vi "Main.vi"(8 "error in (no error)":errorcluster, 11 "Stop notifier":refnum<notifier>) -> (0 "error out":errorcluster)   [LabVIEW 2017, in "Error.lvlib"]
doc: "Module main"
uses:
  Error.lvlib
  ctl/StateData.ctl
  ctl/MainStates.ctl
  ctl/ErrorInfo.ctl
  <vilib>/ErrorRing/Error Ring.xnode
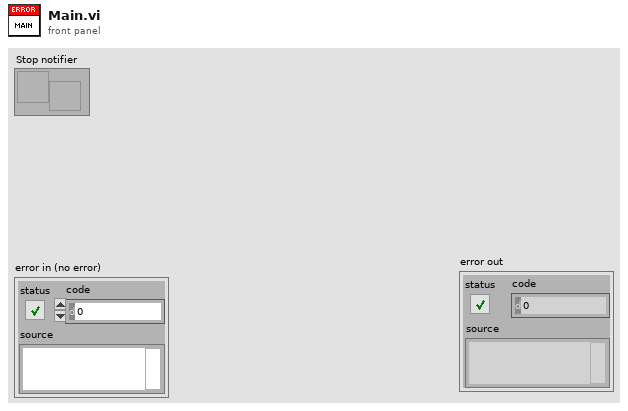
[diagram p1: front panel]
types:
  T1 = typedef "Error.lvlib/StateData.ctl" = cluster{"Blank":dbl}
  T2 = typedef "Error.lvlib/ErrorInfo.ctl" = cluster{"error in":errorcluster, "Text":string, "From":string, "Kill":bool}
  T3 = typedef "Error.lvlib/MainStates.ctl" = enum16{"Timeout", "Error", "Exit", "Init", "ClassError", "LogError", "Shutdown", "Warning"}
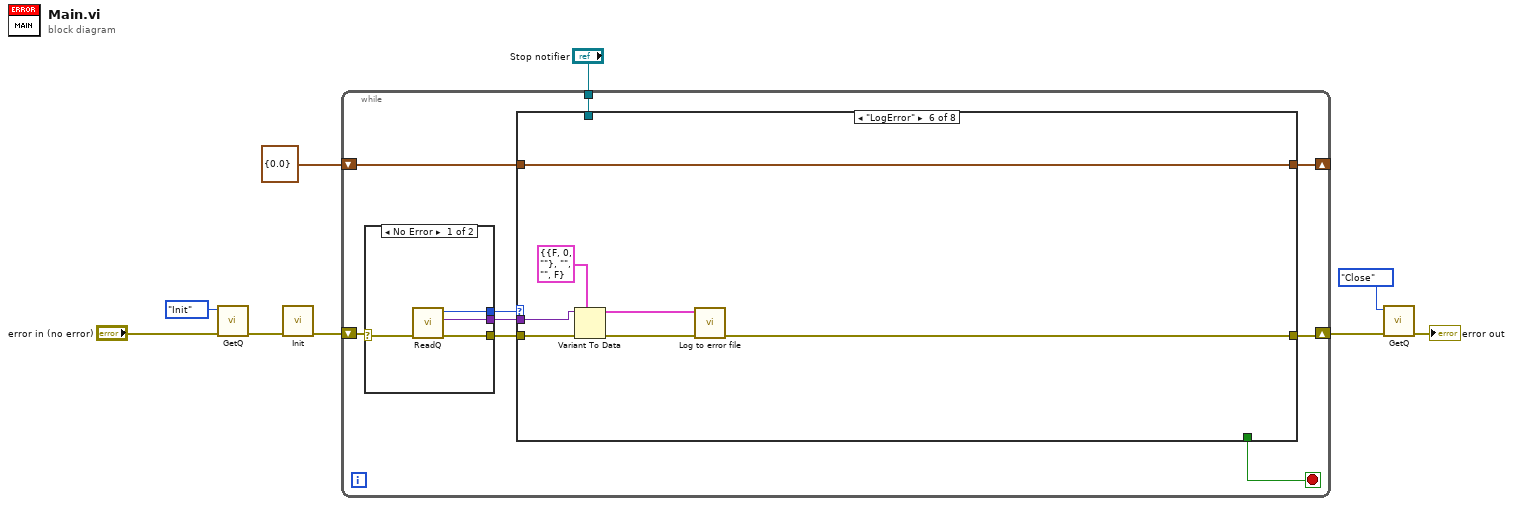
[diagram p0: block diagram]
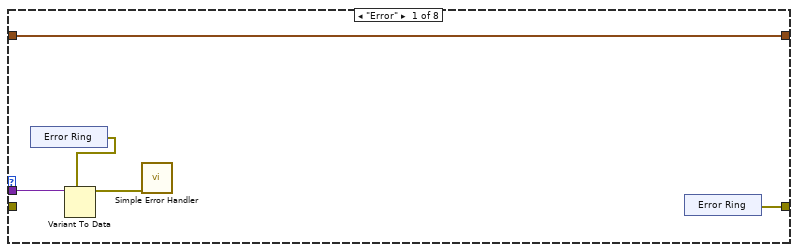
[diagram p2: hidden frame]
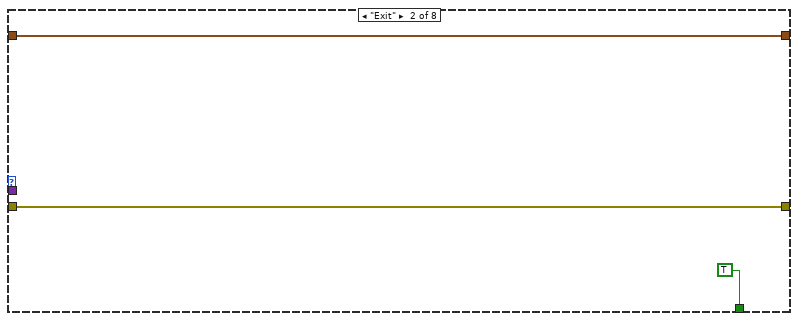
[diagram p3: hidden frame]
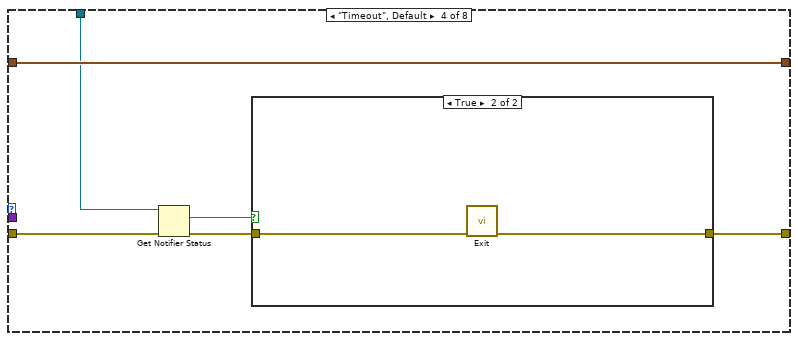
[diagram p5: hidden frame]
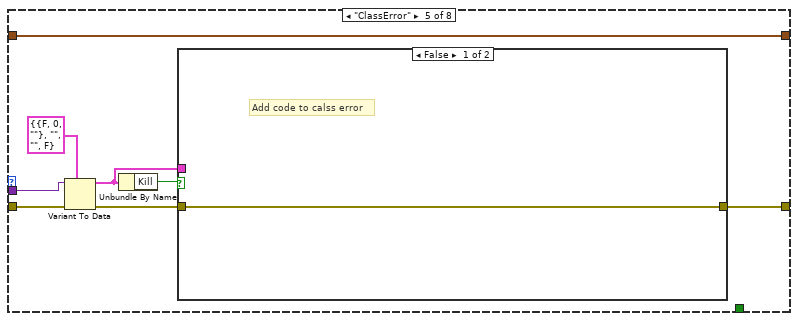
[diagram p7: hidden frame]
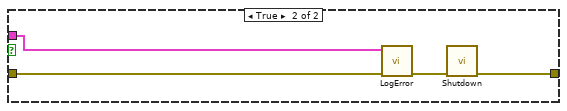
[diagram p8: hidden frame]
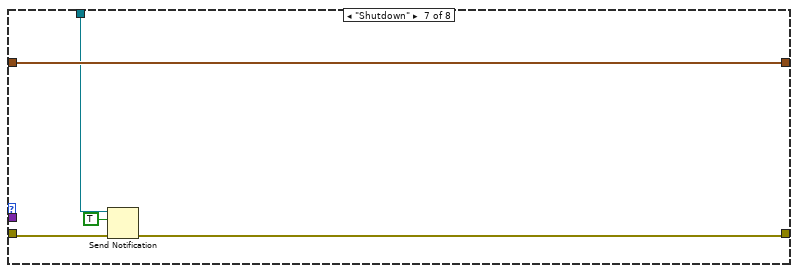
[diagram p9: hidden frame]
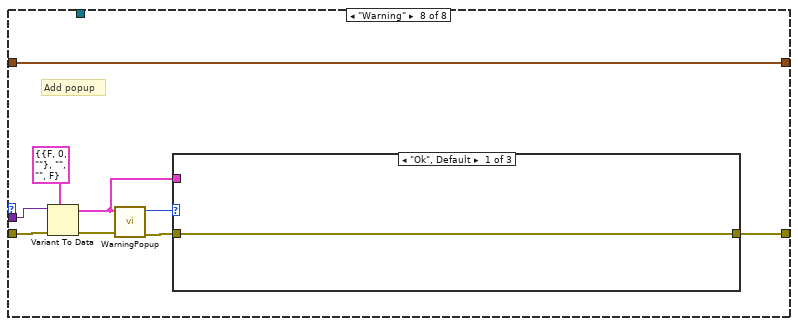
[diagram p10: hidden frame]
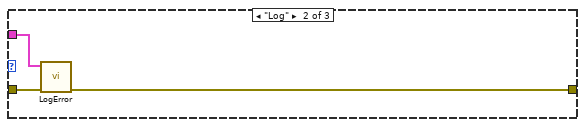
[diagram p11: hidden frame]
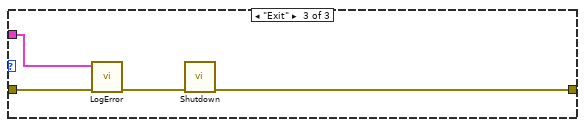
[diagram p12: hidden frame]
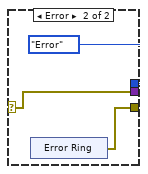
[diagram p13: hidden frame]
diagram:
  n1 = call "GetQ.vi"("error in (no error)"="error in (no error)", "Mode (Get)"=enum16{"Get", "Close", "Init"}."Init") -> ("error out"=w2:errorcluster)  [unwired: 8 in, 1 out]
  n2 = call "Init.vi"("error in (no error)"=w2) -> ("error out"=w1:errorcluster)  [unwired: 10 in]
  n3 = while {
    shift-right: [w14] -> w6
    shift-left: w1 -> [w18]
    shift-right: [w11] -> _
    shift-left: T1 {"Blank"=0.0} ("Cluster") -> [w12]
    tunnel: "Stop notifier" -> [w10]
    stop <- w13 stop-if-true
    n4 = case shown="No Error" w18 {
      selector: w18 -> [w85 w87]
      tunnel: [w84 MainStates."Error" ("State")] -> w17
      tunnel: [w83 w87] -> w16
      tunnel: [w82 w86] -> w15
      frame No Error {
        n5 = call "ReadQ.vi"("error in (no error)"=w85) -> ("error out"=w82:errorcluster, "Variant"=w83:variant, "State"=w84:T3)  [unwired: 8 in]
      }
      frame Error {
        n6 = xnode "Error Ring"() -> ("error out"=w86:errorcluster)
      }
    }
    n7 = case shown="\"LogError\"" w17 {
      tunnel: w16 -> [w23 _ _ _ w45 w56 _ w71]
      tunnel: w15 -> [_ w28 w30 w35 w46 w57 w63 w70]
      tunnel: [w22 w28 w30 w32 w41 w54 w60 w65] -> w14
      tunnel: [_ TRUE _ _ _ _ _ _] -> w13
      tunnel: w12 -> [w19 w26 w29 w36 w47 w59 w64 w73]
      tunnel: [w19 w26 w29 w36 w47 w59 w64 w73] -> w11
      tunnel: w10 -> [_ _ _ w34 _ _ w62 _]
      frame "Error" {
        n8 = xnode "Error Ring"() -> ("error out"=w21:errorcluster)
        n9 = Variant To Data(type=w21, Variant=w23) -> (data=w20:errorcluster)  [unwired: 1 in, 1 out]
        n10 = call <vilib>:"Simple Error Handler.vi"("error in (no error)"=w20) -> ()  [unwired: 4 in, 5 out]
        n11 = xnode "Error Ring"() -> ("error out"=w22:errorcluster)
      }
      frame "Exit" {
      }
      frame "Init" {
      }
      frame "Timeout", Default {
        n12 = Get Notifier Status(notifier=w34, error in (no error)=w35) -> (current notification=w33:bool, error out=w31:errorcluster)  [unwired: 3 out]
        n13 = case shown="True" w33 {
          tunnel: [w37 w38] -> w32
          tunnel: w31 -> [w37 w39]
          frame False {
          }
          frame True {
            n14 = call "Exit.vi"("error in (no error)"=w39) -> ("error out"=w38:errorcluster)  [unwired: 10 in]
          }
        }
      }
      frame "ClassError" {
        n15 = Variant To Data(error in=w46, type=T2 {"error in"={"status"=FALSE, "code"=0, "source"=""}, "Text"="", "From"="", "Kill"=FALSE} ("Error info"), Variant=w45) -> (data=w40:T2, error out=w42:errorcluster)
        n16 = Unbundle By Name(w40) -> ("Kill"=w43:bool)
        n17 = case shown="False" w43 {
          tunnel: w42 -> [w48 w50]
          tunnel: [w48 w52] -> w41
          tunnel: w40 -> [_ w49]
          frame False {
            # "Add code to calss error"
          }
          frame True {
            n18 = call "LogError.vi"("error in (no error)"=w50, "Error info"=w49) -> ("error out"=w51:errorcluster)  [unwired: 9 in]
            n19 = call "Shutdown.vi"("error in (no error)"=w51) -> ("error out"=w52:errorcluster)  [unwired: 10 in]
          }
        }
      }
      frame "LogError" {
        n20 = Variant To Data(error in=w57, type=T2 {"error in"={"status"=FALSE, "code"=0, "source"=""}, "Text"="", "From"="", "Kill"=FALSE} ("Error info"), Variant=w56) -> (data=w53:T2, error out=w55:errorcluster)
        n21 = call "Log to error file.vi"("error in (no error)"=w55, "Error info"=w53) -> ("error out"=w54:errorcluster)  [unwired: 9 in]
      }
      frame "Shutdown" {
        n22 = Send Notification(notification=TRUE, notifier=w62, error in (no error)=w63) -> (error out=w60:errorcluster)  [unwired: 1 out]
      }
      frame "Warning" {
        # "Add popup"
        n23 = Variant To Data(error in=w70, type=T2 {"error in"={"status"=FALSE, "code"=0, "source"=""}, "Text"="", "From"="", "Kill"=FALSE} ("Error info"), Variant=w71) -> (data=w66:T2, error out=w69:errorcluster)
        n24 = call "WarningPopup.vi"("error in (no error)"=w69, "Error info"=w66) -> ("error out"=w67:errorcluster, "Select"=w68:enum16{"Ok", "Log", "Exit"})  [unwired: 8 in]
        n25 = case shown="\"Ok\", Default" w68 {
          tunnel: w67 -> [w74 w77 w81]
          tunnel: w66 -> [_ w76 w80]
          tunnel: [w74 w75 w78] -> w65
          frame "Ok", Default {
          }
          frame "Log" {
            n26 = call "LogError.vi"("error in (no error)"=w77, "Error info"=w76) -> ("error out"=w75:errorcluster)  [unwired: 9 in]
          }
          frame "Exit" {
            n27 = call "LogError.vi"("error in (no error)"=w81, "Error info"=w80) -> ("error out"=w79:errorcluster)  [unwired: 9 in]
            n28 = call "Shutdown.vi"("error in (no error)"=w79) -> ("error out"=w78:errorcluster)  [unwired: 10 in]
          }
        }
      }
    }
  }
  n29 = call "GetQ.vi"("error in (no error)"=w6, "Mode (Get)"=enum16{"Get", "Close", "Init"}."Close") -> ("error out"=→"error out":errorcluster)  [unwired: 8 in, 1 out]
